vi "Start Sync.vi"(8 "error in (no error)":errorcluster, 10 "MeasurementPlugin in":refnum<class "MeasurementPluginService.lvclass">, 11 "MeasurementServiceV1 in":refnum<class "MeasurementServiceV1.lvclass">) -> (0 "error out":errorcluster, 3 "MeasurementServiceV1 out":refnum<class "MeasurementServiceV1.lvclass">)   [LabVIEW 2020, in "MeasurementLink Measurement Server.lvlib" / "MeasurementServiceV1.lvclass"]
uses:
  MeasurementServiceV1.lvclass
  MeasurementPluginService/MeasurementPluginService.lvclass
  MeasurementServiceV1.lvclass/MeasurementServiceV1.ctl
  MeasurementLink Measurement Server Internal/RPC Service/MeasurementService/MeasurementService.lvclass/MeasurementService.ctl
  MeasurementLink Measurement Server Internal/RPC Service/MeasurementService/Accessor/Read Server RPC Methods.vi
  MeasurementLink Measurement Server Internal/RPC Service/MeasurementService/MeasurementService.lvclass
  C:/Program Files/National Instruments/LabVIEW 2020/vi.lib/gRPC/LabVIEW gRPC Servicer/ServiceBase/ServiceBase.lvclass
  IMeasurementService/IMeasurementService.lvclass
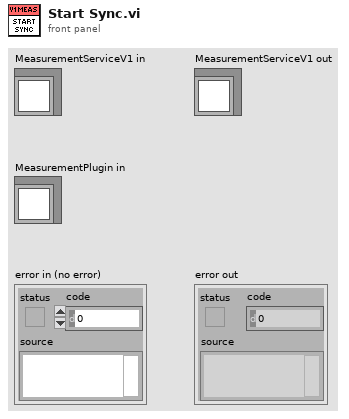
[diagram p1: front panel]
types:
  T1 = typedef "MeasurementLink Measurement Server Internal.lvlib/MeasurementService.lvclass/Server gRPC UEs.ctl" = cluster{"MeasurementService GetMetadata gRPC UE":refnum<user-event>, "MeasurementService Measure gRPC UE":refnum<user-event>}
  T2 = typedef "grpc-lvsupport-release.lvlib/grpcId.ctl" = u64
  T3 = typedef "MeasurementLink Measurement Server.lvlib/GetMetadataResponse.ctl" = cluster{"measurement_details":T4, "measurement_signature":T5, "user_interface_details":T11[]}
  T4 = typedef "MeasurementLink Measurement Server.lvlib/MeasurementDetails.ctl" = cluster{"display_name":string, "version":string}
  T5 = typedef "MeasurementLink Measurement Server.lvlib/MeasurementSignature.ctl" = cluster{"configuration_parameters_message_type":string, "configuration_parameters":T6[], "configuration_defaults":T8, "outputs_message_type":string, "outputs":T9[]}
  T6 = typedef "MeasurementLink Measurement Server.lvlib/ConfigurationParameter.ctl" = cluster{"field_number":i32, "type":i32, "name":string, "repeated":bool, "annotations":T7[]}
  T7 = typedef "MeasurementLink Measurement Server.lvlib/ConfigurationParameter_AnnotationsEntry.ctl" = cluster{"key":string, "value":string}
  T8 = typedef "grpc-lvsupport-release.lvlib/Any.ctl" = cluster{"Type Url":string, "Bytes":u8[]}
  T9 = typedef "MeasurementLink Measurement Server.lvlib/Output.ctl" = cluster{"field_number":i32, "type":i32, "name":string, "repeated":bool, "annotations":T10[]}
  T10 = typedef "MeasurementLink Measurement Service V2.lvlib/ni_measurementlink_measurement_v2_Output_AnnotationsEntry.ctl" = cluster{"key":string, "value":string}
  T11 = typedef "MeasurementLink Measurement Server.lvlib/UserInterfaceDetails.ctl" = cluster{"file_url":string}
  T12 = typedef "MeasurementLink Measurement Server Internal.lvlib/ni_measurementlink_measurement_v1_GetMetadataResponse.ctl" = cluster{"measurement_details":T13, "measurement_signature":T14, "user_interface_details":T19[]}
  T13 = typedef "MeasurementLink Measurement Server Internal.lvlib/ni_measurementlink_measurement_v1_MeasurementDetails.ctl" = cluster{"display_name":string, "version":string}
  T14 = typedef "MeasurementLink Measurement Server Internal.lvlib/ni_measurementlink_measurement_v1_MeasurementSignature.ctl" = cluster{"configuration_parameters_message_type":string, "configuration_parameters":T15[], "configuration_defaults":T17, "outputs_message_type":string, "outputs":T18[]}
  T15 = typedef "MeasurementLink Measurement Server Internal.lvlib/ni_measurementlink_measurement_v1_ConfigurationParameter.ctl" = cluster{"field_number":i32, "type":i32, "name":string, "repeated":bool, "annotations":T16[]}
  T16 = typedef "MeasurementLink Measurement Server Internal.lvlib/ni_measurementlink_measurement_v1_ConfigurationParameter_AnnotationsEntry.ctl" = cluster{"key":string, "value":string}
  T17 = typedef "MeasurementLink Measurement Server Internal.lvlib/google_protobuf_Any.ctl" = cluster{"type_url":string, "value":u8[]}
  T18 = typedef "MeasurementLink Measurement Server Internal.lvlib/ni_measurementlink_measurement_v1_Output.ctl" = cluster{"field_number":i32, "type":i32, "name":string, "repeated":bool}
  T19 = typedef "MeasurementLink Measurement Server Internal.lvlib/ni_measurementlink_measurement_v1_UserInterfaceDetails.ctl" = cluster{"file_url":string}
  T20 = typedef "MeasurementLink Measurement Server Internal.lvlib/ni_measurementlink_measurement_v1_MeasureRequest.ctl" = cluster{"configuration_parameters":T17, "pin_map_context":T21}
  T21 = typedef "MeasurementLink Measurement Server Internal.lvlib/ni_measurementlink_PinMapContext.ctl" = cluster{"pin_map_id":string, "sites":i32[]}
  T22 = typedef "MeasurementLink Measurement Server.lvlib/MeasureResponse.ctl" = cluster{"outputs":T17}
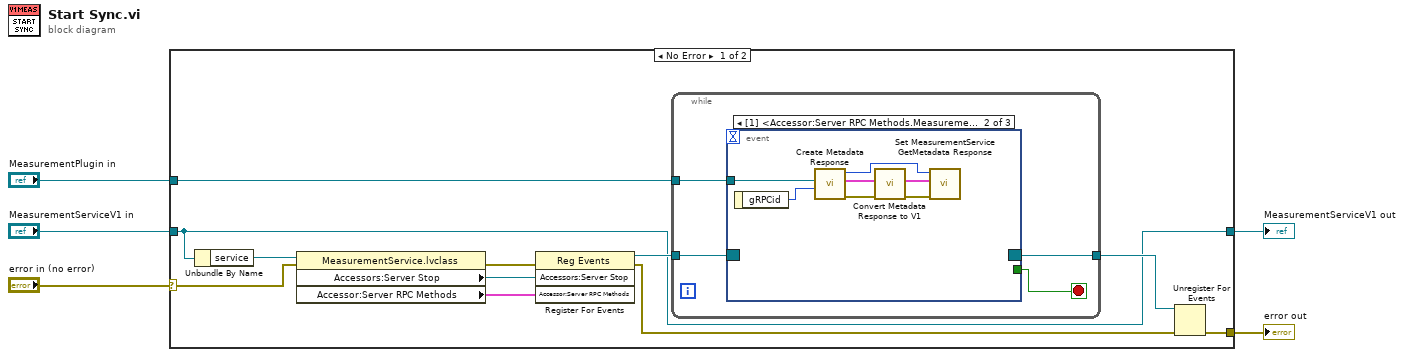
[diagram p0: block diagram]
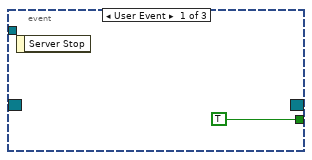
[diagram p2: hidden frame]
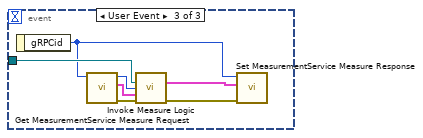
[diagram p3: hidden frame]
diagram:
  n1 = case shown="No Error" "error in (no error)" {
    selector: "error in (no error)" -> [w10 w37]
    tunnel: [w14 w37] -> w3
    tunnel: "MeasurementPlugin in" -> [w11 _]
    tunnel: "MeasurementServiceV1 in" -> [w7 w36]
    tunnel: [w7 w36] -> w1
    frame No Error {
      n2 = Unbundle By Name(w7) -> ("service"=w13:refnum<class "MeasurementService.lvclass">)
      n3 = property class="MeasurementService.lvclass"(reference=w13, error in=w10) -> (error out=w9:errorcluster, "Accessors:Server Stop"=w12:refnum<user-event>, "Accessor:Server RPC Methods"=w8:T1)  [unwired: 1 out]
      n4 = register-events(error in=w9, w12, w8) -> (reference out=w16:refnum<event-registration>, error out=w6:errorcluster)  [unwired: 1 in]
      n5 = while {
        tunnel: w16 -> [w20]
        tunnel: [w19] -> w15
        tunnel: w11 -> [w18]
        stop <- w17 stop-if-true
        n6 = event "RPC Methods Event Structure" shown="[1] <Accessor:Server RPC Methods.MeasurementService GetMetadata gRPC UE>: User Event" {
          selector: w20 -> [_ _ _]
          dyn-events: [_ _ _] -> w19
          timeout: _ -> [_ _ _]
          tunnel: [TRUE _ _] -> w17
          tunnel: w18 -> [_ w26 w34]
          event User Event {
            n7 = event-data() -> ()  [unwired: 1 in, 1 out]
          }
          event User Event {
            n8 = event-data() -> ("gRPCid"=w27:T2)  [unwired: 1 in]
            n9 = call "Create Metadata Response.vi"("gRPCid"=w27, "MeasurementPluginService in"=w26) -> ("error out"=w25:errorcluster, "Get Metadata Response"=w23:T3, "gRPCid out"=w28:T2)  [unwired: 7 in]
            n10 = call "Convert Metadata Response to V1.vi"("error in (no error)"=w25, "GetMetadataResponse Generic in"=w23) -> ("error out"=w24:errorcluster, "GetMetadataResponse V1 out"=w22:T12)  [unwired: 8 in]
            n11 = call "Set MeasurementService GetMetadata Response.vi"("error in (no error)"=w24, "Message Data"=w22, "gRPCid in"=w28) -> ()  [unwired: 8 in, 1 out]
          }
          event User Event {
            n12 = event-data() -> ("gRPCid"=w31:T2)  [unwired: 1 in]
            n13 = call "Get MeasurementService Measure Request.vi"("gRPCid in"=w31) -> ("error out"=w32:errorcluster, "Message Data"=w29:T20, "gRPCid out"=w30:T2)  [unwired: 8 in]
            n14 = call "Invoke Measure Logic.vi"("MeasurementPlugin in"=w34, "gRPCid in"=w30, "MeasureRequest"=w29, "error in (no error)"=w32) -> ("Measure Response"=w33:T22, "error out"=w35:errorcluster)  [unwired: 10 in]
            n15 = call "Set MeasurementService Measure Response.vi"("error in (no error)"=w35, "Message Data"=w33, "gRPCid in"=w31) -> ()  [unwired: 8 in, 1 out]
          }
        }
      }
      n16 = Unregister For Events(event registration refnum=w15, error in=w6) -> (error out=w14:errorcluster)
    }
    frame Error {
    }
  }
  "error out" <- w3
  "MeasurementServiceV1 out" <- w1
